vi "query.vi"(0 "pallet number":i16, 1 "pallet_num sel":bool, 2 "TIME":u16(ring) items=["selected period", "last day", "last week", "last mounth", "Last Turn"], 3 "time select":bool, 4 "FROM":timestamp, 5 "UNTIL":timestamp, 6 "GB_SITUATION":u16(ring) items=["normal", "warning", "error"], 7 "GB_sit sel":bool, 8 "DEFECTS_TYPE":u16(ring) items=["1", "2"], 9 "CURV_SITUATION":u16(ring) items=["normal", "error"], 10 "def_type sel":bool, 11 "curv_sit sel":bool, 12 "SWR":u16(ring) items=["normal", "error"], 13 "SWL":u16(ring) items=["normal", "error"], 14 "SWR sel":bool, 15 "swl sel":bool, 16 "Pallet-sit":u16(ring) items=["normal", "warning", "error"], 17 "database name":string="PALLETCAR", 18 "pallet_sit sel":bool, 24 "table name":string="pallet", 25 "error in (no error)":errorcluster) -> (20 "Table":string[][](table), 27 "error out 2":errorcluster)   [LabVIEW 2019]
uses:
  <vilib>/addons/database/Connection.llb/DB Tools Open Connec (String).vi
  <vilib>/addons/database/_DB Variant To Data/Database Variant To Data.xnode
  <vilib>/addons/database/NI_Database_API.lvlib
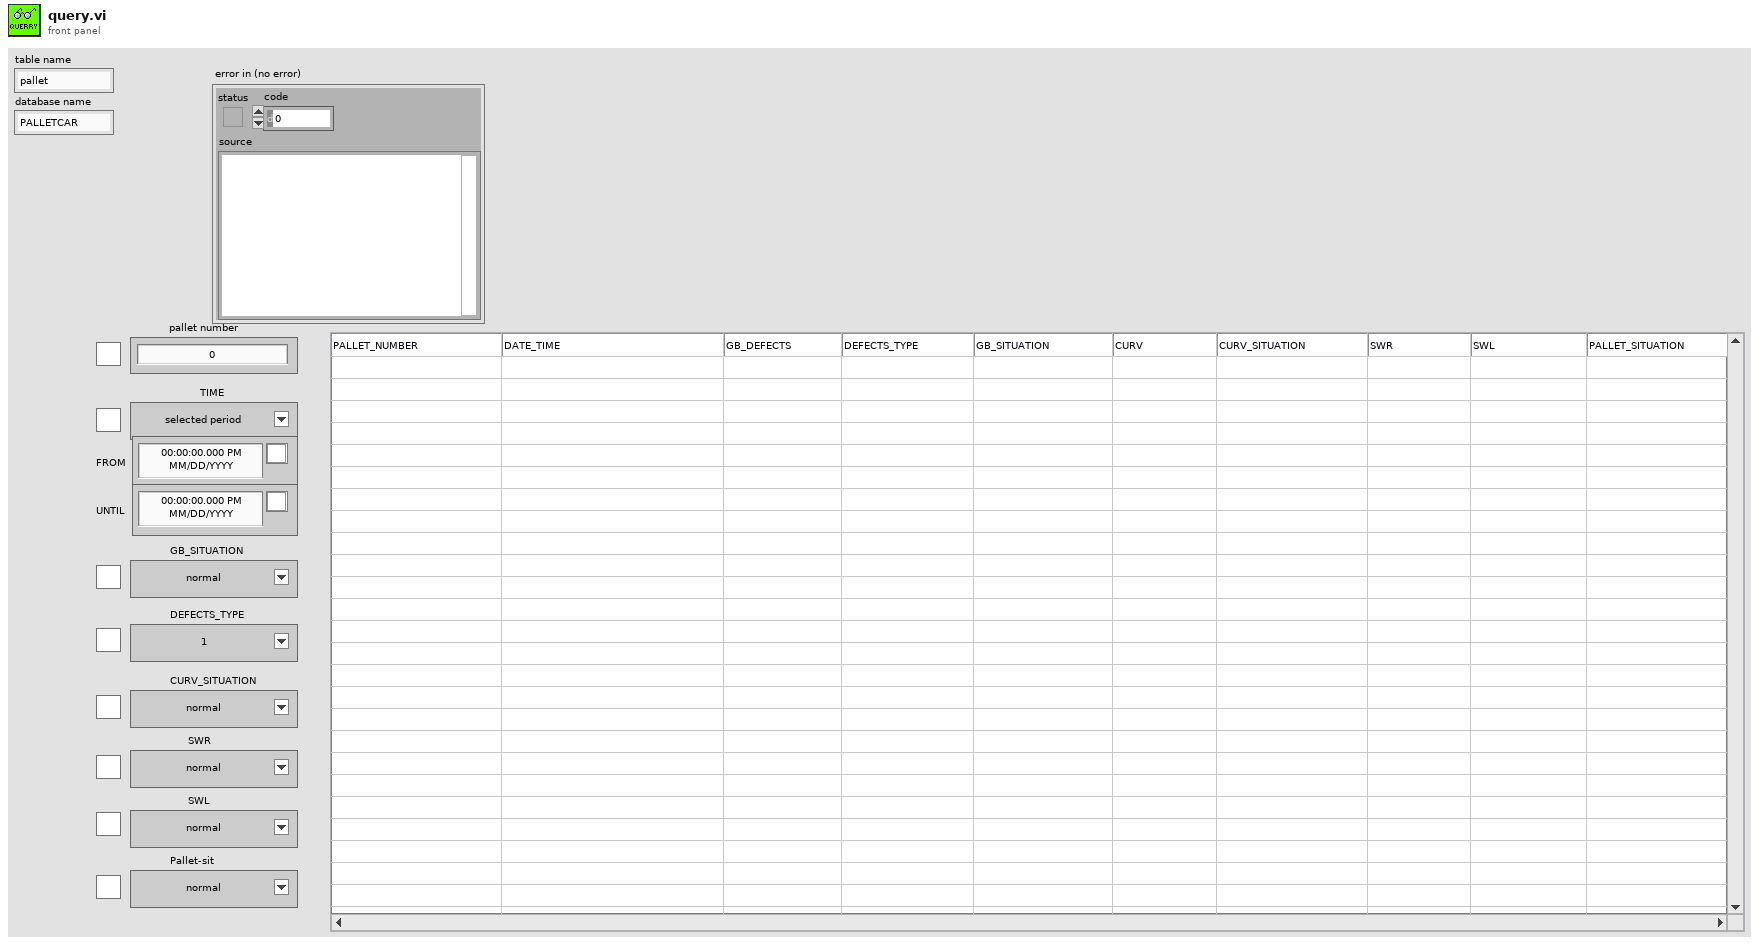
[diagram p1: front panel]
types:
  T1 = typedef "NI_Database_API.lvlib/Conn ObjectReference.ctl" = refnum<k1>
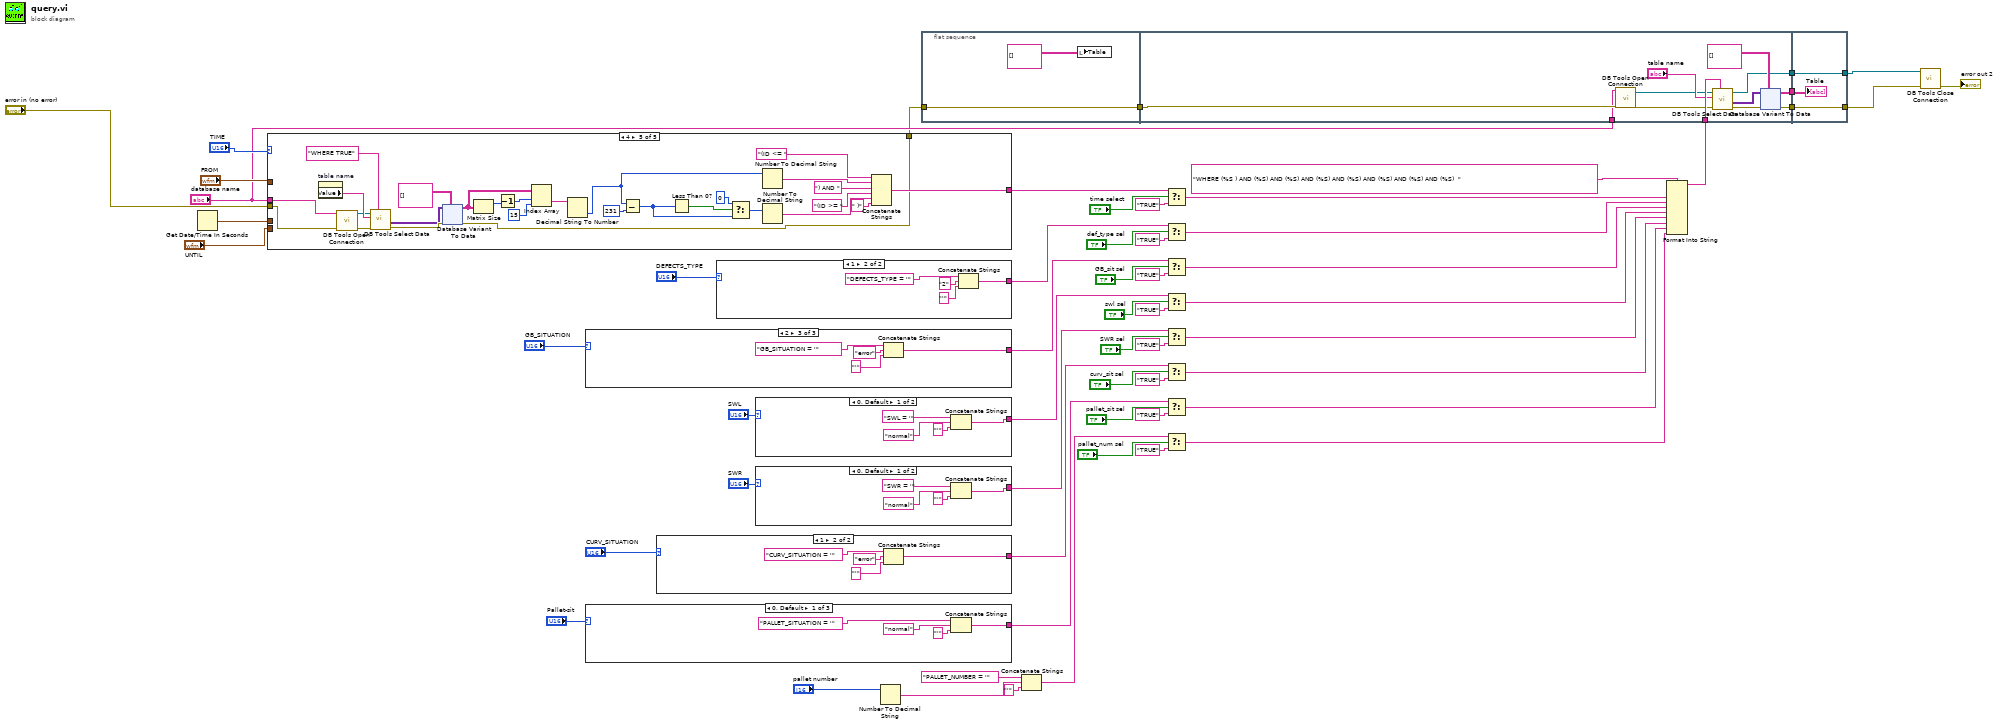
[diagram p0: block diagram]
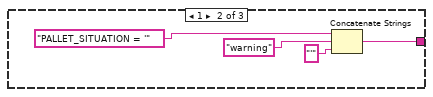
[diagram p2: hidden frame]
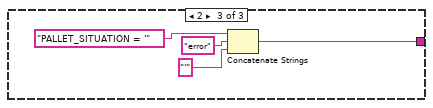
[diagram p3: hidden frame]
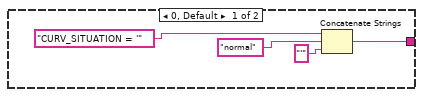
[diagram p4: hidden frame]
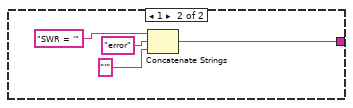
[diagram p5: hidden frame]
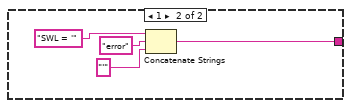
[diagram p6: hidden frame]
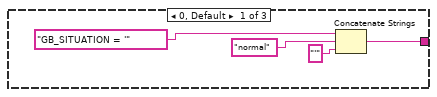
[diagram p7: hidden frame]
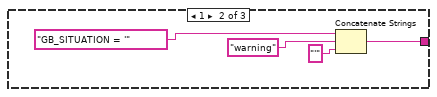
[diagram p8: hidden frame]
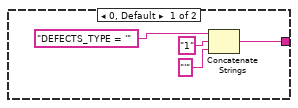
[diagram p9: hidden frame]
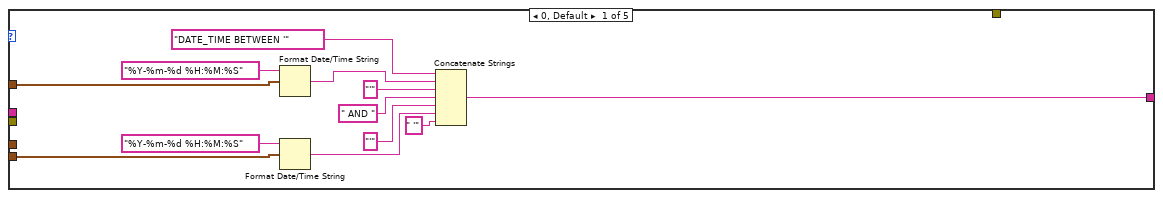
[diagram p10: hidden frame]
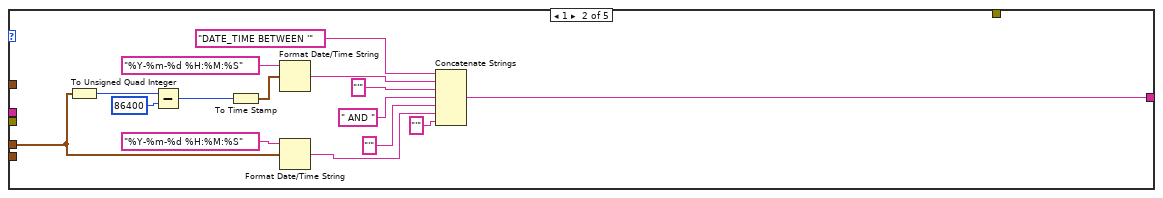
[diagram p11: hidden frame]
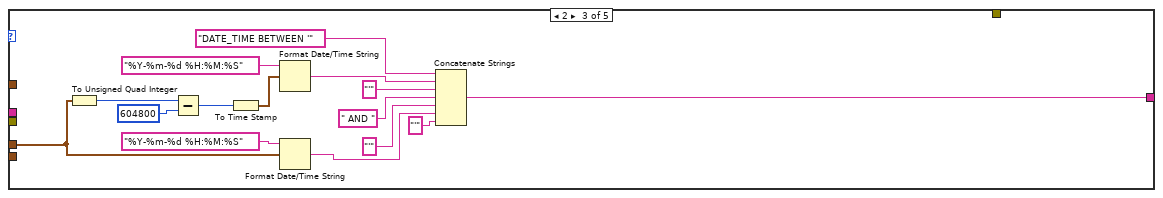
[diagram p12: hidden frame]
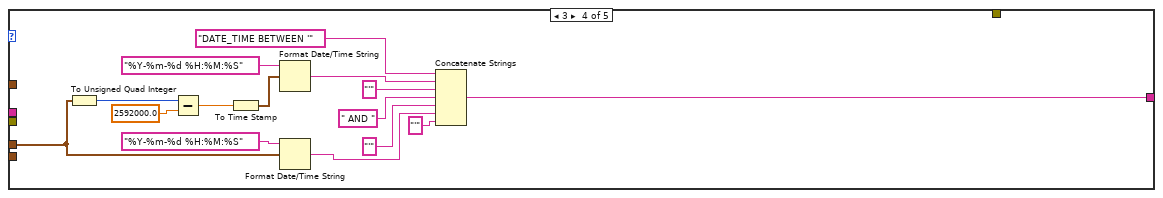
[diagram p13: hidden frame]
diagram:
  n1 = Get Date/Time In Seconds() -> (seconds since 1Jan1904=w48:timestamp)
  n2 = case shown="4" "TIME" {
    tunnel: "FROM" -> [w67 _ _ _ _]
    tunnel: "UNTIL" -> [w65 _ _ _ _]
    tunnel: [w60 w75 w86 w101 w127] -> w21
    tunnel: w48 -> [_ w73 w88 w103 _]
    tunnel: "error in (no error)" -> [_ _ _ _ w119]
    tunnel: [_ _ _ _ w120] -> w1
    tunnel: "database name" -> [_ _ _ _ w116]
    frame 0, Default {
      n3 = Format Date/Time String(time format string (%c)="%Y-%m-%d %H:%M:%S", seconds (now)=w67) -> (date/time string=w66:string)  [unwired: 1 in]
      n4 = Format Date/Time String(time format string (%c)="%Y-%m-%d %H:%M:%S", seconds (now)=w65) -> (date/time string=w62:string)  [unwired: 1 in]
      n5 = Concatenate Strings("DATE_TIME BETWEEN '" ("condition"), w66, "'" ("string"), " AND " ("time format string (%c)"), "'" ("string"), w62, " '" ("string")) -> (w60:string)
    }
    frame 1 {
      n6 = To Unsigned Quad Integer(1:w73) -> (0:w83:u64)
      n7 = Subtract(x=w83, y=u64 86400) -> (x-y=w85:u64)
      n8 = To Time Stamp(1:w85) -> (0:w74:timestamp)
      n9 = Format Date/Time String(time format string (%c)="%Y-%m-%d %H:%M:%S", seconds (now)=w74) -> (date/time string=w79:string)  [unwired: 1 in]
      n10 = Format Date/Time String(time format string (%c)="%Y-%m-%d %H:%M:%S", seconds (now)=w73) -> (date/time string=w76:string)  [unwired: 1 in]
      n11 = Concatenate Strings("DATE_TIME BETWEEN '" ("condition"), w79, "'" ("string"), " AND " ("time format string (%c)"), "'" ("string"), w76, "'" ("string")) -> (w75:string)
    }
    frame 2 {
      n12 = To Unsigned Quad Integer(1:w88) -> (0:w91:u64)
      n13 = Subtract(x=w91, y=u64 604800) -> (x-y=w89:u64)
      n14 = To Time Stamp(1:w89) -> (0:w87:timestamp)
      n15 = Format Date/Time String(time format string (%c)="%Y-%m-%d %H:%M:%S", seconds (now)=w87) -> (date/time string=w96:string)  [unwired: 1 in]
      n16 = Format Date/Time String(time format string (%c)="%Y-%m-%d %H:%M:%S", seconds (now)=w88) -> (date/time string=w93:string)  [unwired: 1 in]
      n17 = Concatenate Strings("DATE_TIME BETWEEN '" ("condition"), w96, "'" ("condition"), " AND " ("time format string (%c)"), "'" ("string"), w93, "'" ("string")) -> (w86:string)
    }
    frame 3 {
      n18 = To Unsigned Quad Integer(1:w103) -> (0:w105:u64)
      n19 = Subtract(x=w105, y=2592000.0) -> (x-y=w106:dbl)
      n20 = To Time Stamp(1:w106) -> (0:w102:timestamp)
      n21 = Format Date/Time String(time format string (%c)="%Y-%m-%d %H:%M:%S", seconds (now)=w102) -> (date/time string=w111:string)  [unwired: 1 in]
      n22 = Format Date/Time String(time format string (%c)="%Y-%m-%d %H:%M:%S", seconds (now)=w103) -> (date/time string=w114:string)  [unwired: 1 in]
      n23 = Concatenate Strings("DATE_TIME BETWEEN '" ("condition"), w111, "'" ("condition"), " AND " ("time format string (%c)"), "'" ("string"), w114, "'" ("string")) -> (w101:string)
    }
    frame 4 {
      n24 = property on="table name" class="Str"() -> ("Value"=w143:string)  [unwired: 2 in, 2 out]
      n25 = call-poly <vilib>:"DB Tools Open Connection.vi"("error in (no error)"=w119, "connection information"=w116) -> ("error out"=w117:errorcluster, "connection reference"=w118:T1)  [unwired: 6 in]
      n26 = call <vilib>:"DB Tools Select Data.vi"("condition"="WHERE TRUE" ("format string"), "error in (no error)"=w117, "table"=w143, "connection reference"=w118) -> ("error out"=w142:errorcluster, "data"=w141:variant[][])  [unwired: 2 in, 1 out]
      n27 = xnode "Database Variant To Data"("database variant"=w141, "error in (no error)"=w142, "type"=string[][] []) -> ("data"=w126:string[][], "error out"=w120:errorcluster)
      n28 = Matrix Size(0:w126) -> (1:w125:i32)  [unwired: 1 out]
      n29 = Decrement(x=w125) -> (x-1=w124:i32)
      n30 = Index Array(array=w126, index (row)=w124, index (col)=15 ("disabled index (col)")) -> (element=w122:string)
      n31 = Decimal String To Number(string=w122) -> (number=w121:i32)  [unwired: 2 in, 1 out]
      n32 = Subtract(x=w121, y=231) -> (x-y=w136:i32)
      n33 = Less Than 0?(x=w136) -> (x < 0?=w135:bool)
      n34 = Select(t=0 ("y"), s=w135, f=w136) -> (s? t:f=w137:i32)
      n35 = Number To Decimal String(number=w121) -> (decimal integer string=w134:string)  [unwired: 1 in]
      n36 = Number To Decimal String(number=w137) -> (decimal integer string=w138:string)  [unwired: 1 in]
      n37 = Concatenate Strings("(ID <= " ("condition"), w134, ") AND " ("string"), "(ID >= " ("string"), w138, " )" ("string")) -> (w127:string)
    }
  }
  n38 = case shown="2" "GB_SITUATION" {
    tunnel: [w188 w192 w196] -> w35
    frame 0, Default {
      n39 = Concatenate Strings("GB_SITUATION = '" ("string"), "normal" ("string"), "'" ("string")) -> (w188:string)
    }
    frame 1 {
      n40 = Concatenate Strings("GB_SITUATION = '" ("string"), "warning" ("string"), "'" ("string")) -> (w192:string)
    }
    frame 2 {
      n41 = Concatenate Strings("GB_SITUATION = '" ("string"), "error" ("string"), "'" ("string")) -> (w196:string)
    }
  }
  n42 = case shown="0, Default" "Pallet-sit" {
    tunnel: [w200 w204 w208] -> w27
    frame 0, Default {
      n43 = Concatenate Strings("PALLET_SITUATION = '" ("string"), "normal" ("string"), "'" ("string")) -> (w200:string)
    }
    frame 1 {
      n44 = Concatenate Strings("PALLET_SITUATION = '" ("string"), "warning" ("string"), "'" ("string")) -> (w204:string)
    }
    frame 2 {
      n45 = Concatenate Strings("PALLET_SITUATION = '" ("string"), "error" ("string"), "'" ("string")) -> (w208:string)
    }
  }
  n46 = case shown="1" "CURV_SITUATION" {
    tunnel: [w212 w216] -> w29
    frame 0, Default {
      n47 = Concatenate Strings("CURV_SITUATION = '" ("string"), "normal" ("string"), "'" ("string")) -> (w212:string)
    }
    frame 1 {
      n48 = Concatenate Strings("CURV_SITUATION = '" ("string"), "error" ("string"), "'" ("string")) -> (w216:string)
    }
  }
  n49 = case shown="1" "DEFECTS_TYPE" {
    tunnel: [w220 w224] -> w42
    frame 0, Default {
      n50 = Concatenate Strings("DEFECTS_TYPE = '" ("string"), "1" ("string"), "'" ("string")) -> (w220:string)
    }
    frame 1 {
      n51 = Concatenate Strings("DEFECTS_TYPE = '" ("string"), "2" ("string"), "'" ("string")) -> (w224:string)
    }
  }
  n52 = case shown="0, Default" "SWL" {
    tunnel: [w228 w232] -> w33
    frame 0, Default {
      n53 = Concatenate Strings("SWL = '" ("string"), "normal" ("string"), "'" ("string")) -> (w228:string)
    }
    frame 1 {
      n54 = Concatenate Strings("SWL = '" ("string"), "error" ("string"), "'" ("string")) -> (w232:string)
    }
  }
  n55 = case shown="0, Default" "SWR" {
    tunnel: [w236 w240] -> w31
    frame 0, Default {
      n56 = Concatenate Strings("SWR = '" ("string"), "normal" ("string"), "'" ("string")) -> (w236:string)
    }
    frame 1 {
      n57 = Concatenate Strings("SWR = '" ("string"), "error" ("string"), "'" ("string")) -> (w240:string)
    }
  }
  n58 = Number To Decimal String(number="pallet number") -> (decimal integer string=w47:string)  [unwired: 1 in]
  n59 = flat-sequence {
    tunnel: [w244] -> w11
    tunnel: w1 -> [w244]
    tunnel: [w255] -> w58
    tunnel: [w253] -> w57
    tunnel: w12 -> [w252]
    tunnel: [w251] -> w56
    tunnel: w11 -> [w249]
    tunnel: "database name" -> [w246]
    tunnel: w56 -> [w303]
    tunnel: w57 -> [w304]
    tunnel: w58 -> [w302]
    tunnel: [w304] -> w6
    tunnel: [w302] -> w5
    frame #0 {
      n60 = local write "Table"(string[][] []) -> ()
    }
    frame #1 {
      n61 = call-poly <vilib>:"DB Tools Open Connection.vi"("error in (no error)"=w249, "connection information"=w246) -> ("error out"=w247:errorcluster, "connection reference"=w248:T1)  [unwired: 6 in]
      n62 = call <vilib>:"DB Tools Select Data.vi"("condition"=w252, "error in (no error)"=w247, "table"="table name", "connection reference"=w248) -> ("error out"=w257:errorcluster, "data"=w256:variant[][], "connection reference out"=w253:T1)  [unwired: 2 in]
      n63 = xnode "Database Variant To Data"("database variant"=w256, "error in (no error)"=w257, "type"=string[][] []) -> ("data"=w251:string[][], "error out"=w255:errorcluster)
    }
    frame #2 {
      "Table" <- w303
    }
  }
  n64 = Concatenate Strings("PALLET_NUMBER = '" ("string"), w47, "'" ("string")) -> (w25:string)
  n65 = Select(t=w21, s="time select", f="TRUE") -> (s? t:f=w20:string)
  n66 = Select(t=w42, s="def_type sel", f="TRUE") -> (s? t:f=w19:string)
  n67 = Select(t=w35, s="GB_sit sel", f="TRUE") -> (s? t:f=w18:string)
  n68 = Select(t=w33, s="swl sel", f="TRUE") -> (s? t:f=w17:string)
  n69 = Select(t=w31, s="SWR sel", f="TRUE") -> (s? t:f=w16:string)
  n70 = Select(t=w29, s="curv_sit sel", f="TRUE") -> (s? t:f=w15:string)
  n71 = Select(t=w27, s="pallet_sit sel", f="TRUE") -> (s? t:f=w14:string)
  n72 = Select(t=w25, s="pallet_num sel", f="TRUE") -> (s? t:f=w13:string)
  n73 = Format Into String(format string="WHERE (%S ) AND (%S) AND (%S) AND (%S) AND (%S) AND (%S) AND (%S) AND (%S)  ", w20, w19, w18, w17, w16, w15, w14, w13) -> (resulting string=w12:string)  [unwired: 2 in, 1 out]
  n74 = call <vilib>:"DB Tools Close Connection.vi"("error in (no error)"=w5, "connection reference"=w6) -> ("error out"=→"error out 2":errorcluster)  [unwired: 5 in]
